vi "题目8.vi"() -> ()   [LabVIEW 2017]
panel:
  in  "x":dbl
  in  "n":dbl
  in  "m":dbl
  out "输出变量 2":dbl
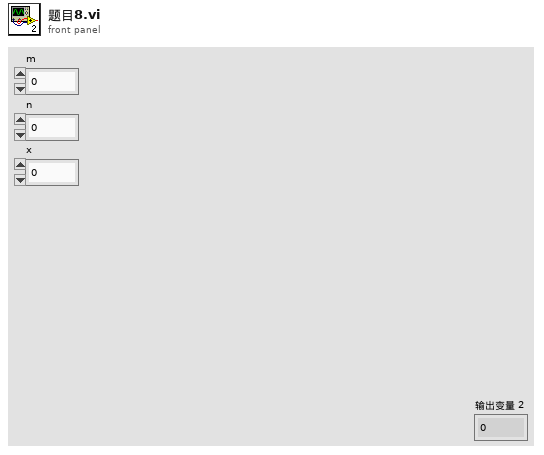
[diagram p1: front panel]
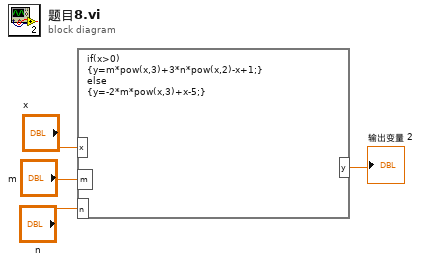
[diagram p0: block diagram]
diagram:
  n1 = formula code="if(x>0)\n{y=m*pow(x,3)+3*n*pow(x,2)-x+1;}\nelse \n{y=-2*m*pow(x,3)+x-5;}"("m"="m", "n"="n", "x"="x") -> ("y"=→"输出变量 2":dbl)
